vi "Replace Item Property.vi"(8 "error in (no error)":errorcluster, 9 "Replace Value":string, 10 "Replace Column":T1, 11 "VI in":refnum<class "VI.lvclass">) -> (0 "error out":errorcluster, 3 "VI out":refnum<class "VI.lvclass">)   [LabVIEW 2020, in "VI Properties Editor.lvlib" / "VI.lvclass"]
doc: "Replaces the value of the property identified by <B>Replace Column</B> with <B>Replace Value</B>."
uses:
  VI.lvclass
  C:/Users/acasalen/Documents/LabVIEW Data/Projects/VI-Properties-Editor/source/Classes/Item/Item.lvclass
  CTLs/Replace Column.ctl
  VI Properties Editor.lvlib
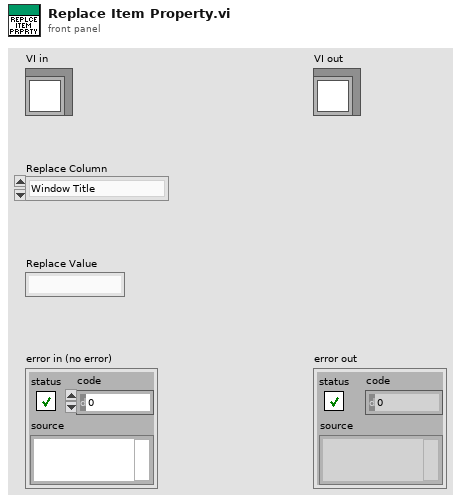
[diagram p1: front panel]
types:
  T1 = typedef "VI Properties Editor.lvlib/Replace Column.ctl" = enum16{"Window Title", "Description", "Help Path", "Help Tag", "Custom Title?", "Help URL", "Help Type", "Control Label", "Control Caption", "Control Description", "Control Tip Strip"}
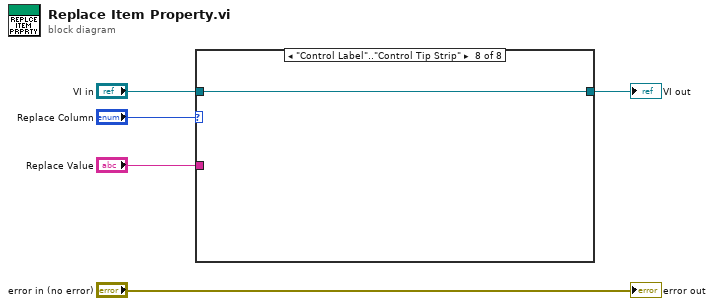
[diagram p0: block diagram]
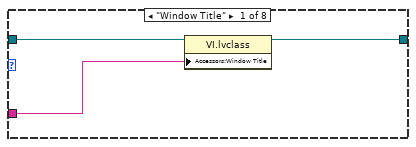
[diagram p2: hidden frame]
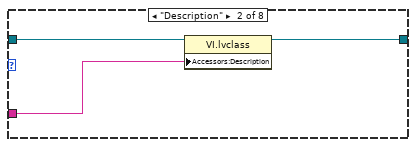
[diagram p3: hidden frame]
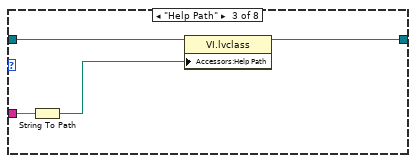
[diagram p4: hidden frame]
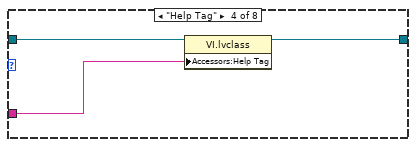
[diagram p5: hidden frame]
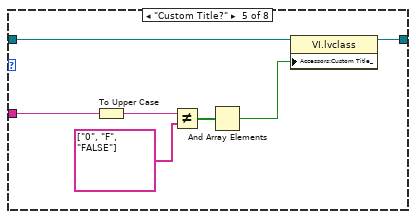
[diagram p6: hidden frame]
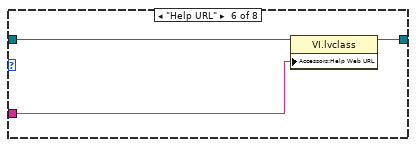
[diagram p7: hidden frame]
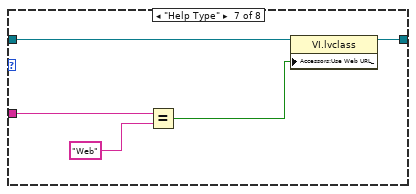
[diagram p8: hidden frame]
diagram:
  n1 = case shown="\"Control Label\"..\"Control Tip Strip\"" "Replace Column" {
    tunnel: "VI in" -> [w8 w11 w15 w18 w25 w28 w33 w34]
    tunnel: [w7 w10 w14 w17 w24 w27 w32 w34] -> w3
    tunnel: "Replace Value" -> [w6 w9 w13 w16 w23 w26 w31 _]
    frame "Window Title" {
      n2 = property class="VI.lvclass"(reference=w8, "Accessors:Window Title"=w6) -> (reference out=w7:refnum<class "VI.lvclass">)  [unwired: 1 in, 1 out]
    }
    frame "Description" {
      n3 = property class="VI.lvclass"(reference=w11, "Accessors:Description"=w9) -> (reference out=w10:refnum<class "VI.lvclass">)  [unwired: 1 in, 1 out]
    }
    frame "Help Path" {
      n4 = String To Path(string=w13) -> (path=w12:path)
      n5 = property class="VI.lvclass"(reference=w15, "Accessors:Help Path"=w12) -> (reference out=w14:refnum<class "VI.lvclass">)  [unwired: 1 in, 1 out]
    }
    frame "Help Tag" {
      n6 = property class="VI.lvclass"(reference=w18, "Accessors:Help Tag"=w16) -> (reference out=w17:refnum<class "VI.lvclass">)  [unwired: 1 in, 1 out]
    }
    frame "Custom Title?" {
      n7 = To Upper Case(1:w23) -> (0:w22:string)
      n8 = Not Equal?(x=w22, y=string[] ["0", "F", "FALSE"]) -> (x != y?=w20:bool[])
      n9 = And Array Elements(Boolean array=w20) -> (logical AND=w19:bool)
      n10 = property class="VI.lvclass"(reference=w25, "Accessors:Custom Title_"=w19) -> (reference out=w24:refnum<class "VI.lvclass">)  [unwired: 1 in, 1 out]
    }
    frame "Help URL" {
      n11 = property class="VI.lvclass"(reference=w28, "Accessors:Help Web URL"=w26) -> (reference out=w27:refnum<class "VI.lvclass">)  [unwired: 1 in, 1 out]
    }
    frame "Help Type" {
      n12 = Equal?(x=w31, y="Web") -> (x = y?=w29:bool)
      n13 = property class="VI.lvclass"(reference=w33, "Accessors:Use Web URL_"=w29) -> (reference out=w32:refnum<class "VI.lvclass">)  [unwired: 1 in, 1 out]
    }
    frame "Control Label".."Control Tip Strip" {
    }
  }
  "VI out" <- w3
  "error out" <- "error in (no error)"
